vi "ncx_len_NC_attrV.vi"(2 "nelems":i32, 3 "nc_type":T1(ring)) -> (1 "size":i32)   [LabVIEW 2016]
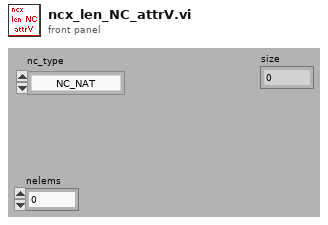
[diagram p1: front panel]
types:
  T1 = enum16{"NC_NAT", "NC_BYTE", "NC_CHAR", "NC_SHORT", "NC_INT", "NC_FLOAT", "NC_DOUBLE"}
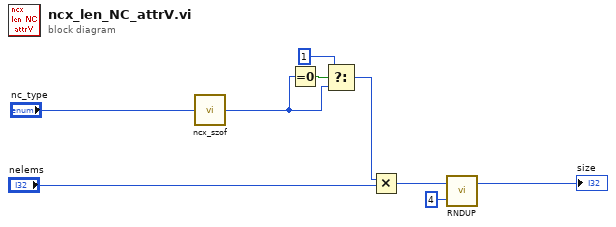
[diagram p0: block diagram]
diagram:
  n1 = call "ncx_szof.vi"("nc_type"="nc_type") -> ("sz"=w3:u64)
  n2 = Equal To 0?(x=w3) -> (x = 0?=w4:bool)
  n3 = Select(t=u64 1, s=w4, f=w3) -> (s? t:f=w2:u64)
  n4 = Multiply(x=w2, y="nelems") -> (x*y=w6:u64)
  n5 = call "RNDUP.vi"("X_ALIGN"=4, "VAR"=w6) -> ("RUDUP"=→"size":i32)  [unwired: 1 out]
